vi "啮合 总回转扭矩.vi"(10 "扭矩反转":dbl[](array[numeric]), 11 "扭矩正转":dbl[](array[numeric])) -> (2 "扭矩反转平均值":dbl, 3 "扭矩正转平均值":dbl)   [LabVIEW 2015, in "Logging.lvlib"]
uses:
  Logging.lvlib
  <vilib>/Analysis/baseanly.llb/Mean (DBL).vi
  <vilib>/Analysis/NI_AALBase.lvlib
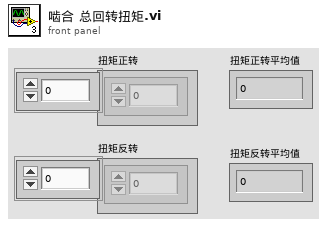
[diagram p1: front panel]
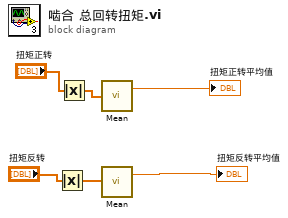
[diagram p0: block diagram]
diagram:
  n1 = Absolute Value(x="扭矩反转") -> (abs(x)=w1:dbl[])
  n2 = Absolute Value(x="扭矩正转") -> (abs(x)=w3:dbl[])
  n3 = call-poly <vilib>:"Mean.vi"("X"=w3) -> ("mean"=→"扭矩正转平均值":dbl)  [unwired: 1 out]
  n4 = call-poly <vilib>:"Mean.vi"("X"=w1) -> ("mean"=→"扭矩反转平均值":dbl)  [unwired: 1 out]
